vi "Initialize--Method.vi"(8 "error in (no error)":errorcluster, 10 "VISA Resource":refnum<visa-resource-name>, 11 "Simulated Thermal Process Controller in":refnum<class "Simulated Thermal Process Controller.lvclass">) -> (0 "error out":errorcluster, 2 "Connected?":bool, 3 "Simulated Thermal Process Controller out":refnum<class "Simulated Thermal Process Controller.lvclass">)   [LabVIEW 2024, in "Simulated Thermal Process Controller.lvclass"]
uses:
  Simulated Thermal Process Controller.lvclass
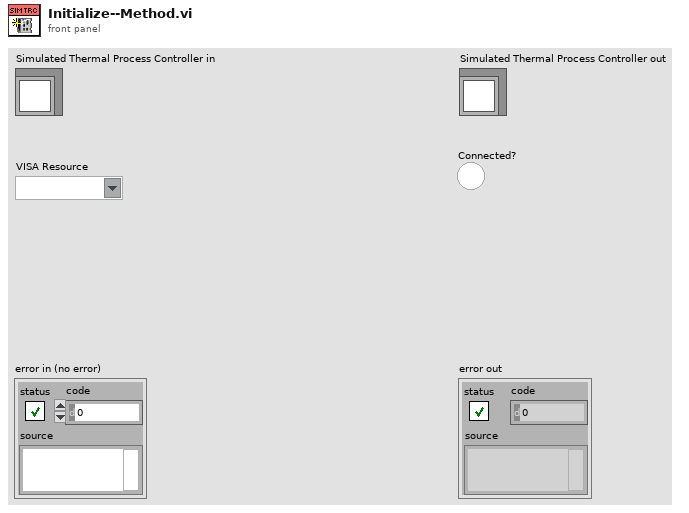
[diagram p1: front panel]
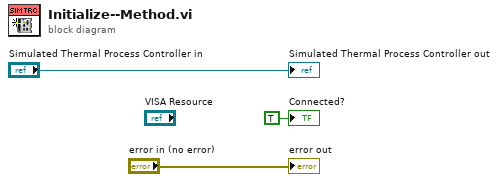
[diagram p0: block diagram]
diagram:
  "error out" <- "error in (no error)"
  "Simulated Thermal Process Controller out" <- "Simulated Thermal Process Controller in"
  "Connected?" <- TRUE ("Connected?")
